vi "ByteArrToHex.vi"(1 "ByteArray":u8[](array[numeric])) -> (0 "HexString":string)   [LabVIEW 2011]
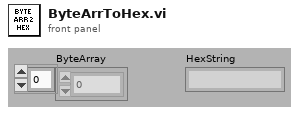
[diagram p1: front panel]
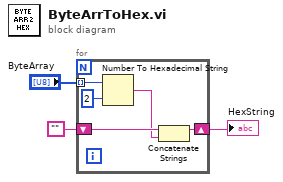
[diagram p0: block diagram]
diagram:
  n1 = for {
    tunnel: "ByteArray" -> [w8] mode=indexing
    shift-right: [w6] -> w3
    shift-left: "" -> [w5]
    n2 = Number To Hexadecimal String(1:i16 2 ("width (-)"), 2:w8) -> (0:w4:string)
    n3 = Concatenate Strings(w5, w4) -> (w6:string)
  }
  "HexString" <- w3
